vi "Periodic Tasks.vi"(8 "error in":errorcluster) -> ()   [LabVIEW 2017]
doc: "This VI runs in parallel to other tasks. It can contain as many user-defined periodic loops as you need. These can carry out PID or other sorts of timed response."
uses:
  <vilib>/Rock Robotics/WPI/ThirdParty/Phoenix-LabVIEW/Motor Controller/Controls/CTRE_Phoenix_MotorControl_ControlMode.ctl
  SwerveLibrary/Drive Motors.ctl
  SwerveLibrary/Swerve Motors.ctl
  Pigeon IMU.ctl
  Arm Control/Arm Motor.ctl
  <vilib>/Rock Robotics/WPI/Solenoid/WPI_SolenoidValue.ctl
  Robot Global Data.vi
  <vilib>/Rock Robotics/Network Tables/NT Write String.vi
  <vilib>/Rock Robotics/WPI/Solenoid/WPI_SolenoidSetEnum.vi
  <vilib>/Rock Robotics/WPI/ThirdParty/Phoenix-LabVIEW/Motor Controller/Get/CTRE_Phoenix_MotorController_GetSelectedSensorData.vi
  <vilib>/addons/control/pid/pid.llb/PID (DBL).vi
  <vilib>/Rock Robotics/Network Tables/NT Write Number.vi
  SwerveLibrary/Huskie Swerve.lvlib
  <vilib>/addons/control/pid/NI_PID_pid.lvlib
  <vilib>/Rock Robotics/Network Tables/NT Read Number.vi
  <vilib>/Rock Robotics/Network Tables/NT Read Boolean.vi
panel:
  out "error out":errorcluster
  in  "Output range":cluster{"output high":dbl, "output low":dbl}={"output high"=1.0, "output low"=-1.0} {"output low" format="%.2f"; "output high" format="%.2f"}
  in  "Shoulder PID":bool=TRUE
  in  "Forearm PID":bool=TRUE
  out "Forearm output":dbl=0.13174219660051584
  out "Shoulder output":dbl=0.06477138484803567
  out "Shoulder angle":dbl=-0.16720390587953488
  out "Elbow angle":dbl=-2.556378983011421
  in  "Forearm PID gains":T1={"proportional gain (Kc)"=0.5, "integral time (Ti, min)"=0.0, "derivative time (Td, min)"=0.0}
  in  "Shoulder PID gains":T1={"proportional gain (Kc)"=1.5, "integral time (Ti, min)"=0.0, "derivative time (Td, min)"=0.0} {"derivative time (Td, min)" format="%.3f"; "integral time (Ti, min)" format="%.3f"; "proportional gain (Kc)" format="%.3f"}
  in  "Forearm Cap":dbl=0.4
  in  "Shoulder Cap":dbl=0.8
  # "Arm Controls"
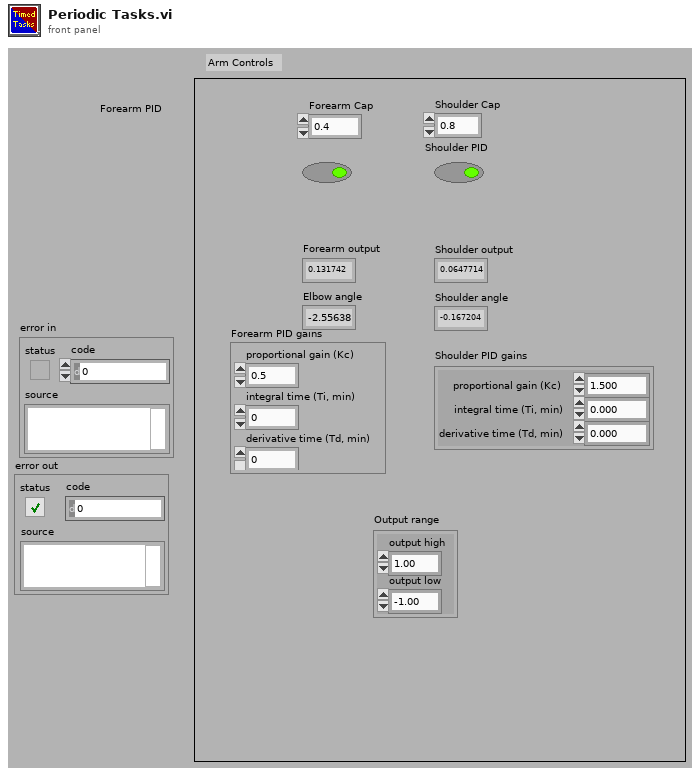
[diagram p1: front panel]
types:
  T1 = cluster{"proportional gain (Kc)":dbl, "integral time (Ti, min)":dbl, "derivative time (Td, min)":dbl}
  T2 = typedef "Pigeon IMU.ctl" = enum16{"Pigeon IMU"}
  T3 = typedef "Huskie Swerve.lvlib/Swerve Motors.ctl" = enum16{"Swerve 1", "Swerve 2", "Swerve 3", "Swerve 4"}
  T4 = typedef "Huskie Swerve.lvlib/Drive Motors.ctl" = enum16{"Drive 1", "Drive 2", "Drive 3", "Drive 4"}
  T5 = typedef "WPI_MotorControlDeviceRef.ctl" = cluster{"DeviceStatus":errorcluster, "Type":T6, "PWM":cluster{"PWM Channel":T7, "DeadBand":T8}, "CAN":cluster{"Device Number":u8, "SetOutput VI Ref":variant, "GetOutput VI Ref":variant, "Enable VI Ref":variant, "Disable VI Ref":variant, "Data":variant}, "Invert":bool, "DIO PWM":cluster{"PWM \"Enable\" Channel":T7, "DIOChannel":T9, "PWM Rate":dbl}}
  T6 = typedef "WPI_MotorControlType.ctl" = enum16{"PWM", "CAN", "DIO PWM"}
  T7 = typedef "FPGA_DIOPWMChannel.ctl" = enum8{"PWM 0", "PWM 1", "PWM 2", "PWM 3", "PWM 4", "PWM 5", "PWM 6", "PWM 7", "PWM 8", "PWM 9", "PWM MXP 0", "PWM MXP 1", "PWM MXP 2", "PWM MXP 3", "PWM MXP 4", "PWM MXP 5", "PWM MXP 6", "PWM MXP 7", "PWM MXP 8", "PWM MXP 9", "Invalid"}
  T8 = typedef "WPI_PWMDeadband.ctl" = cluster{"Name":string, "maxPositivePwm":i32, "minPositivePwm":i32, "centerPwm":i32, "maxNegativePwm":i32, "minNegativePwm":i32, "angularRange":u16}
  T9 = typedef "FPGA_DIOChannel.ctl" = enum8{"DIO 0", "DIO 1", "DIO 2", "DIO 3", "DIO 4", "DIO 5", "DIO 6", "DIO 7", "DIO 8", "DIO 9", "DIO MXP 0", "DIO MXP 1", "DIO MXP 2", "DIO MXP 3", "DIO MXP 4", "DIO MXP 5", "DIO MXP 6", "DIO MXP 7", "DIO MXP 8", "DIO MXP 9", "DIO MXP 10", "DIO MXP 11", "DIO MXP 12", "DIO MXP 13", "DIO MXP 14", "DIO MXP 15", "SPI Port CS1", "SPI Port CS2", "SPI Port CS3", "SPI Port MISO", "SPI Port MOSI", "Invalid"}
  T10 = typedef "CTRE_PigeonIMU_DeviceRef.ctl" = cluster{"DeviceStatus":errorcluster, "Device Number":u8, "Type":T11, "Device ID":u32, "Handle":u64, "UsageFrame":u32, "Library Path":path}
  T11 = typedef "CTRE_PigeonIMU_ConnectionType.ctl" = u32
  T12 = typedef "WPI_DriverStationRobotMode2.ctl" = enum16{"Autonomous Disabled", "Autonomous Enabled", "Teleop Disabled", "Teleop Enabled", "Disconnected", "Finish", "Test Disabled", "Test Enabled", "Emergency Stopped"}
  T13 = cluster{"X":dbl, "Y":dbl, "Z":dbl, "Climber Down":bool, "Climber Up":bool, "X Drive":bool, "Field Relative":bool, "Actuate Grabber":bool, "Inverse Drive":bool}
  T14 = typedef "CTRE_Phoenix_MotorControl_ControlMode.ctl" = u16
  T15 = typedef "WPI_SolenoidValue.ctl" = enum16{"Off", "On", "Forward", "Reverse"}
  T16 = enum16{"Shoulder", "Forearm", "Grabber", "Extra"}[]
  T17 = typedef "Arm Motor.ctl" = enum16{"Shoulder Motor", "Forearm Motor"}
  T18 = typedef "WPI_SolenoidDevRef.ctl" = cluster{"DevStatus":errorcluster, "Pneumatics Control Module":u8, "Forward Solenoid Channel":T19, "Reverse Solenoid Channel":T19}
  T19 = typedef "WPI_SolenoidChannel.ctl" = enum8{"Solenoid 0", "Solenoid 1", "Solenoid 2", "Solenoid 3", "Solenoid 4", "Solenoid 5", "Solenoid 6", "Solenoid 7", "Invalid"}
  T20 = cluster{"Forearm Length":dbl, "Backarm Length":dbl, "Forearm Center of Gravity Length":dbl, "Backarm Center of Gravity Length":dbl, "Weight of Cube":dbl, "Weight of Forearm":dbl, "Weight of Backarm":dbl}
  T21 = cluster{"Forearm importance":dbl, "Backarm importance":dbl}
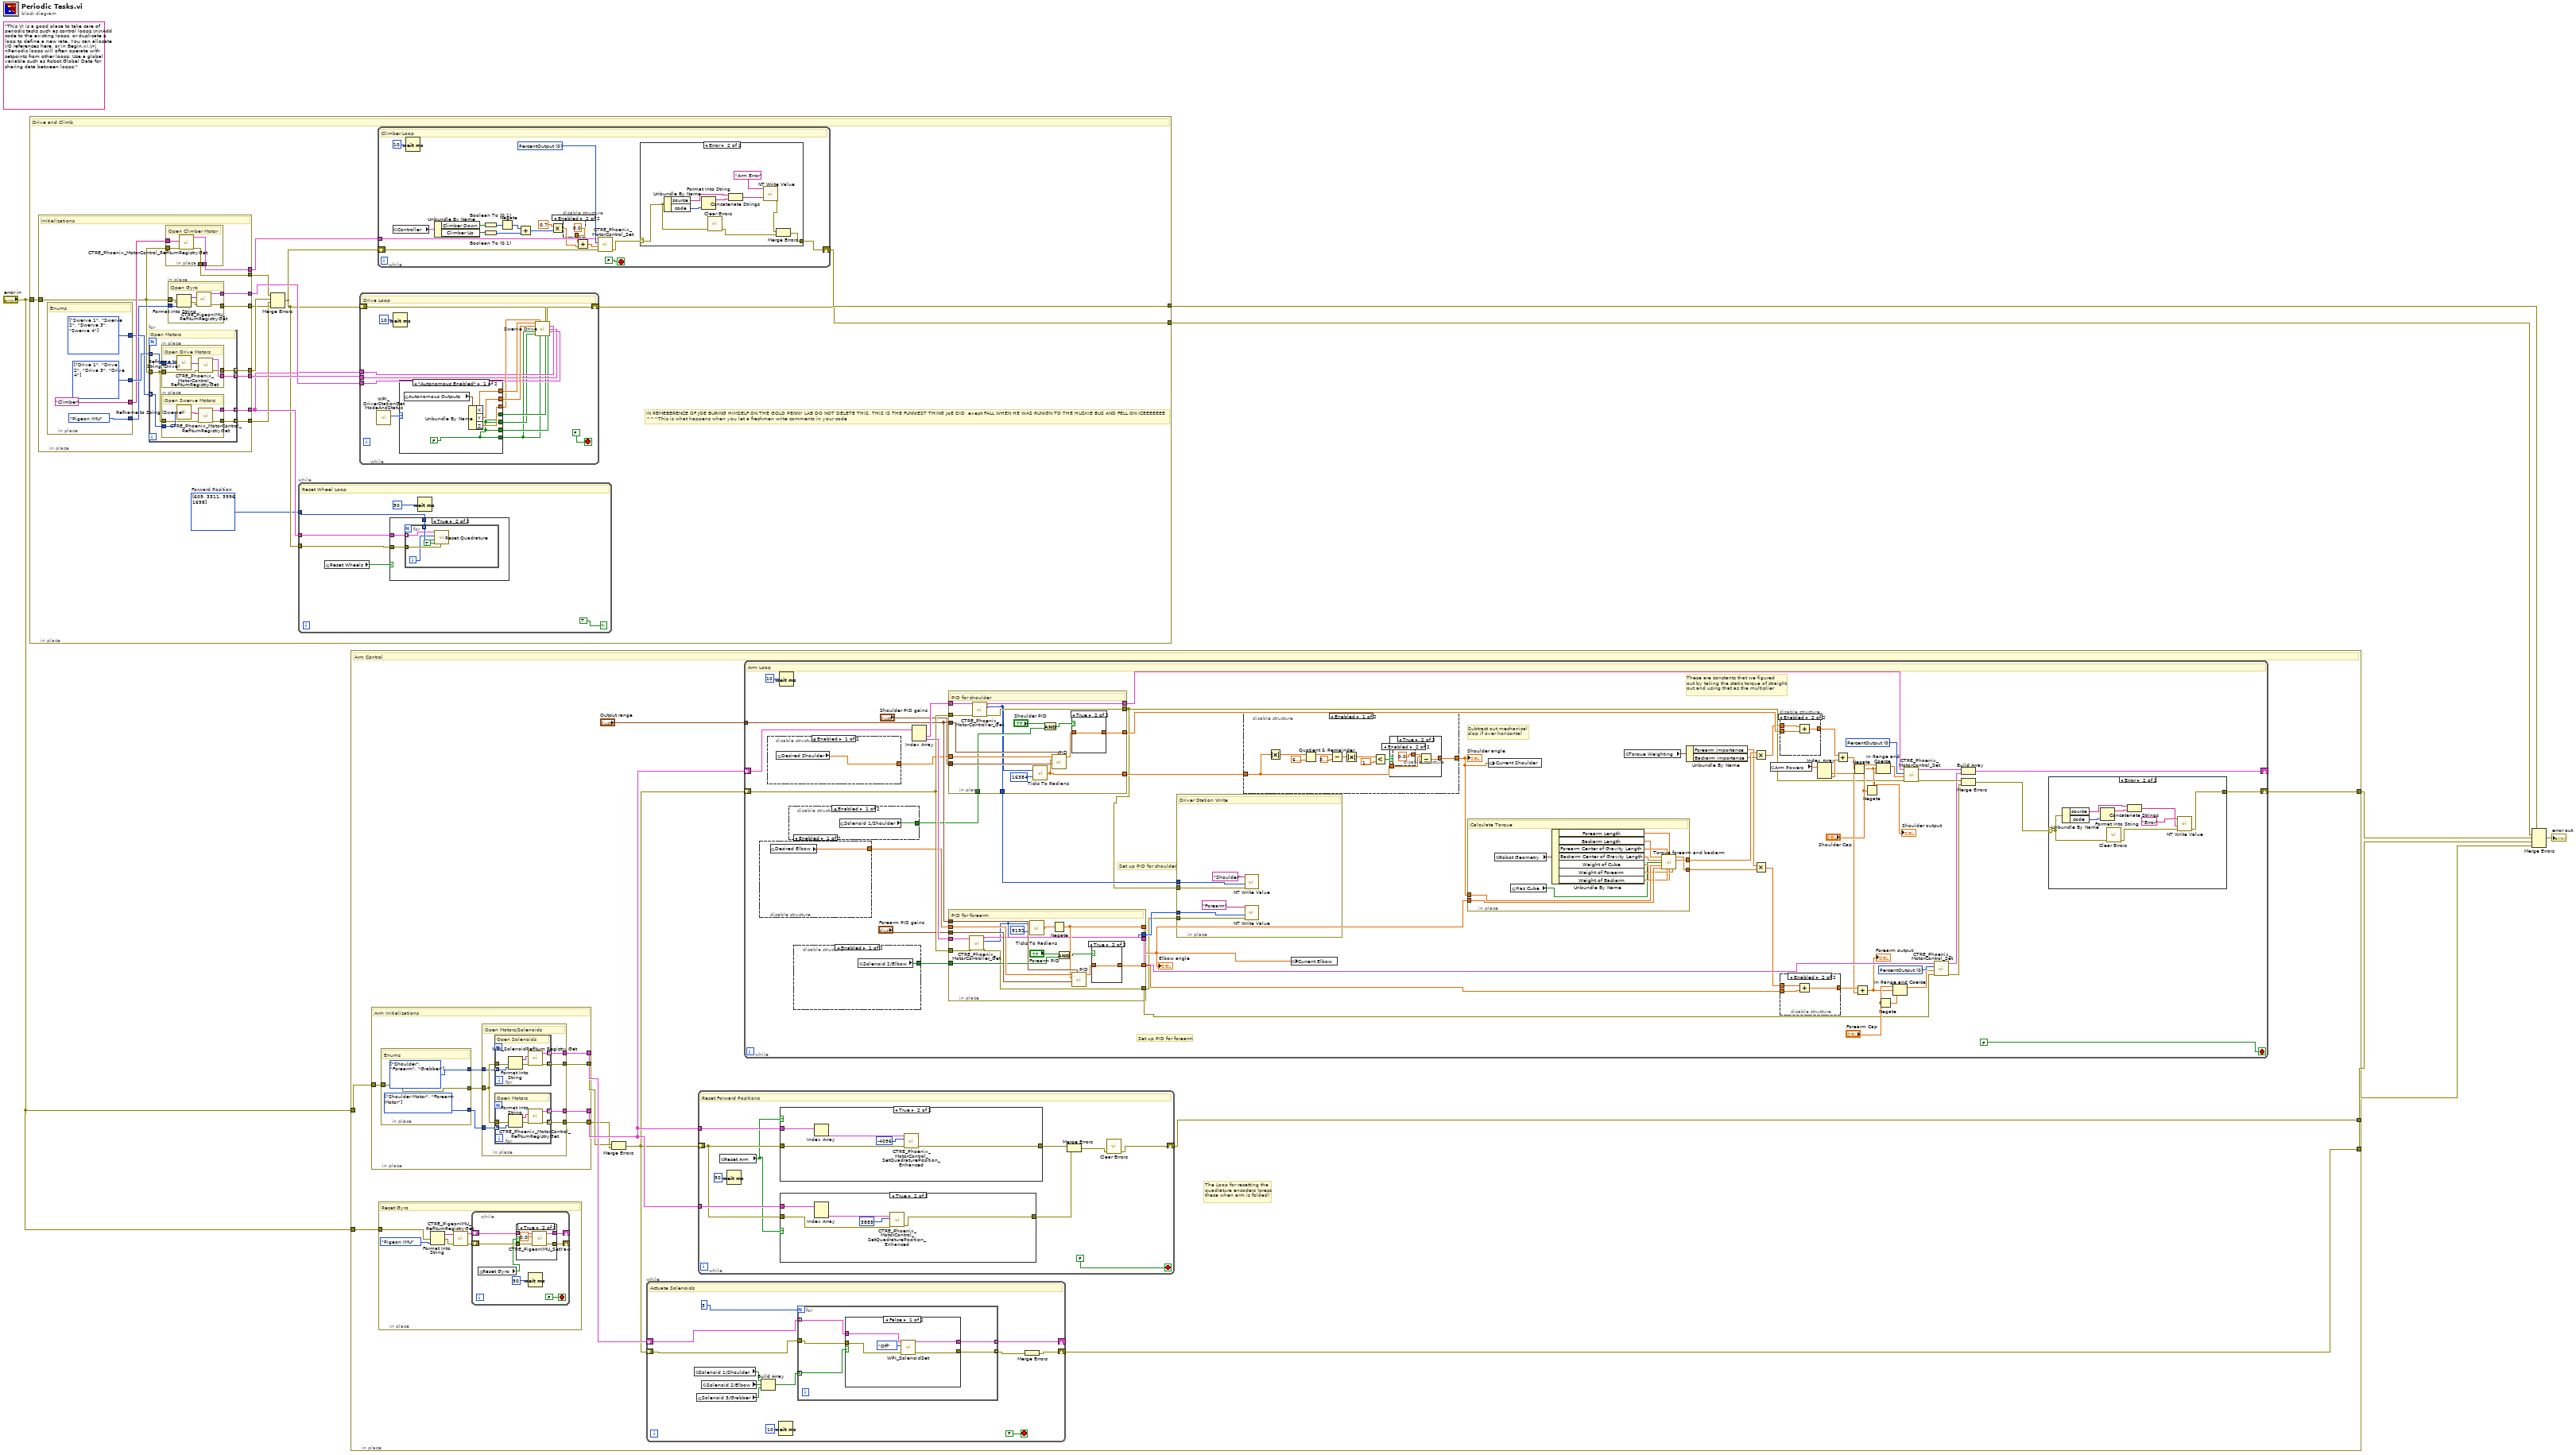
[diagram p0: block diagram]
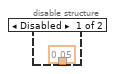
[diagram p3: hidden frame]
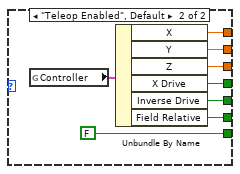
[diagram p5: hidden frame]
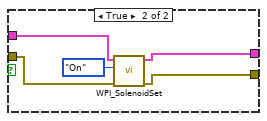
[diagram p7: hidden frame]
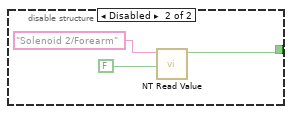
[diagram p10: hidden frame]
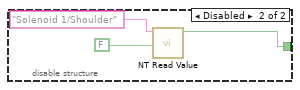
[diagram p11: hidden frame]
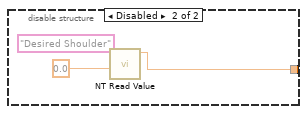
[diagram p12: hidden frame]
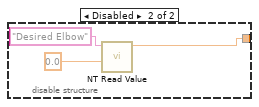
[diagram p13: hidden frame]
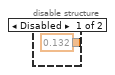
[diagram p16: hidden frame]
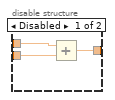
[diagram p18: hidden frame]
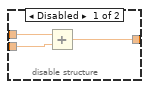
[diagram p19: hidden frame]
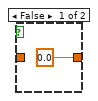
[diagram p20: hidden frame]
diagram:
  (unwired) "This VI is a good place to take care of periodic tasks such as control loops.\n\nAdd code to the existing loops, or duplicate a loop to define a new rate. You can allocate I/O references here, or in Begin.vi.\n\nPeriodic loops will often operate with setpoints from other loops. Use a global variable such as Robot Global Data for sharing data between loops."
  n1 = in-place {
    in-place-border: "error in" -> [w18]
    in-place-border: [w13] -> w7
    in-place-border: [w12] -> w6
    w8 = i32[] [609, 3311, 3996, 1698]  # Forward Position
    # "IN REMEBERENCE OF JOE BURING HIMSELF ON THE GOLD PENNY LAB DO NOT DELETE THIS. THIS IS THE FUNNIEST THING JoE DID  exept FALL WHEN HE WAS RUNIGN TO THE HUSKIE BUS AND FELL ON ICEEEEEEE\n^^^This is what happens when you let a freshmen write comments in your code"
    # "Drive and Climb"
    n2 = in-place {
      in-place-border: [w47] -> w20
      in-place-border: [w46] -> w10
      in-place-border: [w45] -> w19
      in-place-border: [w44] -> w11
      in-place-border: w18 -> [w36]
      in-place-border: [w43] -> w14
      in-place-border: [w42] -> w17
      in-place-border: [w37] -> w16
      in-place-border: [w35] -> w15
      # "Initializations"
      n3 = in-place {
        in-place-border: [w61] -> w41
        in-place-border: ["Climber"] -> w40
        in-place-border: [w59] -> w39
        in-place-border: [Pigeon_IMU."Pigeon IMU" ("Enum")] -> w38
        w59 = T3[] [enum."Swerve 1", enum."Swerve 2", enum."Swerve 3", enum."Swerve 4"] items=["Swerve 1", "Swerve 2", "Swerve 3", "Swerve 4"]
        w61 = T4[] [enum."Drive 1", enum."Drive 2", enum."Drive 3", enum."Drive 4"] items=["Drive 1", "Drive 2", "Drive 3", "Drive 4"]
        # "Enums"
      }
      n4 = for {
        tunnel: w36 -> [w67]
        tunnel: [w68] -> w45 mode=indexing
        tunnel: [w66] -> w47 mode=indexing
        tunnel: [w65] -> w46 mode=indexing
        tunnel: [w64] -> w44 mode=indexing
        tunnel: w41 -> [w63] mode=indexing
        tunnel: w39 -> [w62] mode=indexing
        # "Open Motors"
        n5 = in-place {
          in-place-border: w63 -> [w73]
          in-place-border: [w71] -> w68
          in-place-border: w67 -> [w70]
          in-place-border: [w69] -> w66
          # "Open Drive Motors"
          n6 = call "Refname to String (Drive).vi"("Enum"=w73) -> ("resulting string"=w72:string)
          n7 = call "CTRE_Phoenix_MotorControl_RefNumRegistryGet.vi"("error in (no error)"=w70, "refnum name"=w72) -> ("error out"=w69:errorcluster, "PhoenixMotorControlDevRef"=w71:T5)  [unwired: 8 in]
        }
        n8 = in-place {
          in-place-border: w62 -> [w78]
          in-place-border: w67 -> [w76]
          in-place-border: [w75] -> w65
          in-place-border: [w74] -> w64
          # "Open Swerve Motors"
          n9 = call "Refname to String (Swerve).vi"("Enum"=w78) -> ("String"=w77:string)
          n10 = call "CTRE_Phoenix_MotorControl_RefNumRegistryGet.vi"("error in (no error)"=w76, "refnum name"=w77) -> ("error out"=w75:errorcluster, "PhoenixMotorControlDevRef"=w74:T5)  [unwired: 8 in]
        }
      }
      n11 = in-place {
        in-place-border: w36 -> [w57]
        in-place-border: [w56] -> w43
        in-place-border: [w55] -> w42
        in-place-border: w40 -> [w54]
        # "Open Climber Motor"
        n12 = call "CTRE_Phoenix_MotorControl_RefNumRegistryGet.vi"("error in (no error)"=w57, "refnum name"=w54) -> ("error out"=w56:errorcluster, "PhoenixMotorControlDevRef"=w55:T5)  [unwired: 8 in]
      }
      n13 = in-place {
        in-place-border: w38 -> [w53]
        in-place-border: [w51] -> w37
        in-place-border: w36 -> [w50]
        in-place-border: [w48] -> w35
        # "Open Gyro"
        n14 = Format Into String(error in=w50, w53) -> (resulting string=w52:string, error out=w49:errorcluster)  [unwired: 2 in]
        n15 = call "CTRE_PigeonIMU_RefNumRegistryGet.vi"("error in (no error)"=w49, "refnum name"=w52) -> ("error out"=w48:errorcluster, "PigeonIMUDevRef"=w51:T10)  [unwired: 8 in]
      }
    }
    n16 = Merge Errors(w14, w20, w10, w15) -> (w9:errorcluster)
    n17 = while {
      tunnel: w11 -> [w23]
      tunnel: w9 -> [w25]
      tunnel: w8 -> [w24]
      stop <- TRUE continue-if-true
      # "Reset Wheel Loop"
      n18 = global read "Robot Global Data.vi" "Reset Wheels"() -> (w22:bool)
      n19 = case shown="True" w22 {
        tunnel: w25 -> [_ w29]
        tunnel: w24 -> [_ w28]
        tunnel: w23 -> [_ w27]
        frame False {
        }
        frame True {
          n20 = for {
            tunnel: w29 -> [w34]
            tunnel: w28 -> [w32] mode=indexing
            tunnel: w27 -> [w30] mode=indexing
            i -> [w31]
            n21 = call "Reset Quadrature.vi"("error in"=w34, "Reverse?"=TRUE, "Forward Position"=w32, "Module Number"=w31, "CAN Talon SRX Ref"=w30) -> ()  [unwired: 5 in, 2 out]
          }
        }
      }
      n22 = Wait (ms)(milliseconds to wait=50) -> ()  [unwired: 1 out]
    }
    n23 = while {
      tunnel: w19 -> [w114]
      tunnel: w11 -> [w116]
      tunnel: w16 -> [w115]
      shift-right: [w117] -> w12
      shift-left: w9 -> [w118]
      stop <- FALSE stop-if-true
      # "Drive Loop"
      n24 = call <vilib>:"WPI_DriverStationGetModeAndStatus.vi"() -> ("Robot Mode"=w109:T12)  [unwired: 10 in, 1 out]
      n25 = Wait (ms)(milliseconds to wait=u32 10) -> ()  [unwired: 1 out]
      n26 = case shown="\"Autonomous Enabled\"" w109 {
        tunnel: [w125 w135] -> w121
        tunnel: [w126 w134] -> w120
        tunnel: [w127 w133] -> w119
        tunnel: [w124 w132] -> w113
        tunnel: [w124 w131] -> w112
        tunnel: [w124 w130] -> w111
        tunnel: [w124 FALSE] -> w110
        frame "Autonomous Enabled" {
          w124 = FALSE
          n27 = global read "Robot Global Data.vi" "Autonomous Outputs"() -> (w128:cluster{"X":dbl, "Y":dbl, "Z":dbl})
          n28 = Unbundle By Name(w128) -> ("X"=w125:dbl, "Y"=w126:dbl, "Z"=w127:dbl)
        }
        frame "Teleop Enabled", Default {
          n29 = global read "Robot Global Data.vi" "Controller"() -> (w136:T13)
          n30 = Unbundle By Name(w136) -> ("X"=w135:dbl, "Y"=w134:dbl, "Z"=w133:dbl, "X Drive"=w132:bool, "Inverse Drive"=w130:bool, "Field Relative"=w131:bool)
        }
      }
      n31 = call "Swerve Drive.vi"("X"=w121, "Z"=w119, "error in"=w118, "Y"=w120, "Swerve Dev Ref"=w116, "Drive Dev Ref"=w114, "Straight Drive"=w110, "PigeonIMUDevRef"=w115, "Reverse Drive"=w111, "Low Sensitivity"=w110, "X Drive"=w113, "Field Relative Active"=w112) -> ("error out"=w117:errorcluster)  [unwired: 3 in]
    }
    n32 = while {
      tunnel: w17 -> [w87]
      shift-right: [w82] -> w13
      shift-left: w9 -> [w88]
      stop <- FALSE stop-if-true
      w96 = T14 0 items=["PercentOutput"=0, "Position"=1, "Velocity"=2, "Current"=3, "Follower"=5, "MotionProfile"=6, "MotionMagic"=7, "MotionMagicArc"=8, "MotionProfileArc"=10, "Disabled"=15] ("Control Mode")
      # "Climber Loop"
      n33 = global read "Robot Global Data.vi" "Controller"() -> (w95:T13)
      n34 = Wait (ms)(milliseconds to wait=10) -> ()  [unwired: 1 out]
      n35 = Unbundle By Name(w95) -> ("Climber Down"=w94:bool, "Climber Up"=w93:bool)
      n36 = Boolean To (0,1)(Boolean=w94) -> (0, 1=w92:i16)
      n37 = Boolean To (0,1)(Boolean=w93) -> (0, 1=w90:i16)
      n38 = Negate(x=w92) -> (-x=w91:i16)
      n39 = Add(x=w91, y=w90) -> (x+y=w85:i16)
      n40 = Multiply(x=0.7, y=w85) -> (x*y=w81:dbl)
      n41 = disable-structure shown="Enabled" {
        disable-tunnel: [0.05 0.0] -> w80
        frame Disabled {
        }
        frame Enabled {
        }
      }
      n42 = Add(x=w80, y=w81) -> (x+y=w79:dbl)
      n43 = call "CTRE_Phoenix_MotorControl_Set.vi"("error in (no error)"=w88, "Output"=w79, "Control Mode"=w96, "PhoenixMotorControlDevRef"=w87) -> ("error out"=w83:errorcluster)  [unwired: 6 in, 1 out]
      n44 = case shown="Error" w83 {
        selector: w83 -> [w99 w104]
        tunnel: [w99 w100] -> w82
        frame No Error {
        }
        frame Error {
          n45 = Unbundle By Name(w104) -> ("source"=w106:string, "code"=w108:i32)
          n46 = Format Into String(w108) -> (resulting string=w107:string)  [unwired: 3 in, 1 out]
          n47 = call <vilib>:"Clear Errors.vi"("error in (no error)"=w104) -> ("error out"=w102:errorcluster)  [unwired: 5 in, 1 out]
          n48 = Concatenate Strings(w106, w107) -> (w103:string)
          n49 = call-poly <vilib>:"NT Write Value.vi"("String"=w103, "Name"="Arm Error") -> ("error out"=w101:errorcluster)  [unwired: 9 in]
          n50 = Merge Errors(w101, w102) -> (w100:errorcluster)
        }
      }
    }
  }
  n51 = in-place "In Place Element Structure" {
    in-place-border: "error in" -> [w144]
    in-place-border: [w140] -> w5
    in-place-border: [w139] -> w4
    in-place-border: [w138] -> w3
    in-place-border: "error in" -> [w137]
    # "The Loop for resetting the\nquadrature encoders (press\nthese when arm is folded)"
    # "Arm Control"
    n52 = in-place {
      in-place-border: [w174] -> w142
      in-place-border: [w173] -> w146
      in-place-border: [w172] -> w145
      in-place-border: [w171] -> w143
      in-place-border: w144 -> [w169]
      # "Arm Initializations"
      n53 = in-place {
        in-place-border: [w197] -> w175
        in-place-border: [w196] -> w170
        in-place-border: w169 -> [w195]
        in-place-border: [w195] -> w168
        w196 = T16 [enum."Shoulder", enum."Forearm", enum."Grabber"] items=["Shoulder", "Forearm", "Grabber", "Extra"]
        w197 = T17[] [enum."Shoulder Motor", enum."Forearm Motor"] items=["Shoulder Motor", "Forearm Motor"]
        # "Enums"
      }
      n54 = in-place {
        in-place-border: w175 -> [w182]
        in-place-border: [w181] -> w174
        in-place-border: [w180] -> w173
        in-place-border: [w179] -> w172
        in-place-border: [w178] -> w171
        in-place-border: w168 -> [w177]
        in-place-border: w170 -> [w176]
        # "Open Motors/Solenoids"
        n55 = for {
          tunnel: w176 -> [w194] mode=indexing
          tunnel: w177 -> [w193]
          tunnel: [w190] -> w179 mode=indexing
          tunnel: [w189] -> w178 mode=indexing
          # "Open Solenoids"
          n56 = Format Into String(error in=w193, w194) -> (resulting string=w192:string, error out=w191:errorcluster)  [unwired: 2 in]
          n57 = call <vilib>:"WPI_SolenoidRefNum Registry Get.vi"("error in (no error)"=w191, "refnum name"=w192) -> ("error out"=w189:errorcluster, "SolenoidDevRef"=w190:T18)  [unwired: 8 in]
        }
        n58 = for {
          tunnel: w182 -> [w187] mode=indexing
          tunnel: [w186] -> w180 mode=indexing
          tunnel: [w185] -> w181 mode=indexing
          tunnel: w177 -> [w183]
          # "Open Motors"
          n59 = Format Into String(error in=w183, w187) -> (resulting string=w188:string, error out=w184:errorcluster)  [unwired: 2 in]
          n60 = call "CTRE_Phoenix_MotorControl_RefNumRegistryGet.vi"("error in (no error)"=w184, "refnum name"=w188) -> ("error out"=w185:errorcluster, "PhoenixMotorControlDevRef"=w186:T5)  [unwired: 8 in]
        }
      }
    }
    n61 = in-place "In Place Element Structure" {
      in-place-border: w137 -> [w148]
      # "Reset Gyro"
      n62 = Format Into String(error in=w148, Pigeon_IMU."Pigeon IMU" ("Enum")) -> (resulting string=w152:string, error out=w149:errorcluster)  [unwired: 2 in]
      n63 = call "CTRE_PigeonIMU_RefNumRegistryGet.vi"("error in (no error)"=w149, "refnum name"=w152) -> ("error out"=w151:errorcluster, "PigeonIMUDevRef"=w150:T10)  [unwired: 8 in]
      n64 = while {
        shift-right: [w158] -> _
        shift-left: w150 -> [w159]
        shift-right: [w157] -> _
        shift-left: w151 -> [w160]
        stop <- FALSE stop-if-true
        n65 = global read "Robot Global Data.vi" "Reset Gyro"() -> (w154:bool)
        n66 = case shown="True" w154 {
          tunnel: w160 -> [w161 w167]
          tunnel: w159 -> [w162 w166]
          tunnel: [w162 w164] -> w158
          tunnel: [w161 w163] -> w157
          frame False {
          }
          frame True {
            n67 = call <vilib>:"CTRE_PigeonIMU_SetYaw.vi"("error in (no error)"=w167, "Value"=0.0, "PigeonIMUDevRef"=w166) -> ("error out"=w163:errorcluster, "PigeonIMUDevRef"=w164:T10)  [unwired: 7 in]
          }
        }
        n68 = Wait (ms)(milliseconds to wait=50) -> ()  [unwired: 1 out]
      }
    }
    n69 = Merge Errors(w143, w142) -> (w141:errorcluster)
    n70 = while {
      shift-right: [w203] -> _
      shift-left: w145 -> [w207]
      shift-right: [w198] -> w138
      shift-left: w141 -> [w205]
      stop <- FALSE stop-if-true
      # "Actuate Solenoids"
      n71 = global read "Robot Global Data.vi" "Solenoid 1/Shoulder"() -> (w202:bool)
      n72 = global read "Robot Global Data.vi" "Solenoid 3/Grabber"() -> (w200:bool)
      n73 = global read "Robot Global Data.vi" "Solenoid 2/Elbow"() -> (w201:bool)
      n74 = Build Array(w202, w201, w200) -> (w204:bool[])
      n75 = Wait (ms)(milliseconds to wait=u32 10) -> ()  [unwired: 1 out]
      n76 = for {
        N: 3 -> [_]
        tunnel: w207 -> [w212] mode=indexing
        tunnel: w205 -> [w213]
        tunnel: w204 -> [w214] mode=indexing
        tunnel: [w211] -> w203 mode=indexing
        tunnel: [w210] -> w199 mode=indexing
        n77 = case shown="False" w214 {
          tunnel: w213 -> [w218 w224]
          tunnel: w212 -> [w217 w222]
          tunnel: [w216 w221] -> w211
          tunnel: [w215 w220] -> w210
          frame False {
            n78 = call-poly <vilib>:"WPI_SolenoidSet.vi"("error in (no error)"=w218, "Value"=WPI_SolenoidValue."Off", "SolenoidDevRef"=w217) -> ("error out"=w215:errorcluster, "SolenoidDevRef"=w216:T18)  [unwired: 7 in]
          }
          frame True {
            n79 = call-poly <vilib>:"WPI_SolenoidSet.vi"("error in (no error)"=w224, "Value"=WPI_SolenoidValue."On", "SolenoidDevRef"=w222) -> ("error out"=w220:errorcluster, "SolenoidDevRef"=w221:T18)  [unwired: 7 in]
          }
        }
      }
      n80 = Merge Errors(w199) -> (w198:errorcluster)
    }
    n81 = while {
      tunnel: w146 -> [w233]
      shift-right: [w225] -> w139
      shift-left: w141 -> [w230]
      tunnel: w146 -> [w232]
      stop <- FALSE stop-if-true
      # "Reset Forward Positions"
      n82 = global read "Robot Global Data.vi" "Reset Arm"() -> (w227:bool)
      n83 = Wait (ms)(milliseconds to wait=u32 50) -> ()  [unwired: 1 out]
      n84 = case shown="True" w227 {
        tunnel: w233 -> [_ w246]
        tunnel: w230 -> [w241 w245]
        tunnel: [w241 w243] -> w228
        frame False {
        }
        frame True {
          n85 = Index Array(array=w246) -> (element=w244:T5)  [unwired: 1 in]
          n86 = call <vilib>:"CTRE_Phoenix_MotorControl_SetQuadraturePosition_Enhanced.vi"("error in (no error)"=w245, "New Position"=-4096, "PhoenixMotorControlDevRef"=w244) -> ("error out"=w243:errorcluster)  [unwired: 7 in, 1 out]
        }
      }
      n87 = case shown="True" w227 {
        tunnel: w232 -> [_ w240]
        tunnel: w230 -> [w235 w238]
        tunnel: [w235 w237] -> w229
        frame False {
        }
        frame True {
          n88 = Index Array(array=w240) -> (element #2=w239:T5)  [unwired: 2 in, 1 out]
          n89 = call <vilib>:"CTRE_Phoenix_MotorControl_SetQuadraturePosition_Enhanced.vi"("error in (no error)"=w238, "New Position"=3885, "PhoenixMotorControlDevRef"=w239) -> ("error out"=w237:errorcluster)  [unwired: 7 in, 1 out]
        }
      }
      n90 = Merge Errors(w228, w229) -> (w226:errorcluster)
      n91 = call <vilib>:"Clear Errors.vi"("error in (no error)"=w226) -> ("error out"=w225:errorcluster)  [unwired: 5 in, 1 out]
    }
    n92 = while {
      tunnel: "Output range" -> [w289]
      shift-right: [w291] -> _
      shift-left: w146 -> [w299]
      shift-right: [w249] -> w140
      shift-left: w141 -> [w286]
      stop <- FALSE stop-if-true
      w288 = T14 0 items=["PercentOutput"=0, "Position"=1, "Velocity"=2, "Current"=3, "Follower"=5, "MotionProfile"=6, "MotionMagic"=7, "MotionMagicArc"=8, "MotionProfileArc"=10, "Disabled"=15] ("Control Mode")
      w295 = T14 0 items=["PercentOutput"=0, "Position"=1, "Velocity"=2, "Current"=3, "Follower"=5, "MotionProfile"=6, "MotionMagic"=7, "MotionMagicArc"=8, "MotionProfileArc"=10, "Disabled"=15] ("Control Mode")
      # "Subtract out mechanical\nslop if over horizontal"
      # "Set up PID for shoulder"
      # "These are constants that we figured\nout by taking the static torque of straight\nout and using that as the multiplier"
      # "Set up PID for forearm"
      # "Arm Loop"
      n93 = disable-structure shown="Enabled" {
        disable-tunnel: [w313 w314] -> w281
        frame Enabled {
          n94 = global read "Robot Global Data.vi" "Desired Elbow"() -> (w313:dbl)
        }
        frame Disabled {
          n95 = call-poly <vilib>:"NT Read Value.vi"("Default Value"=0.0, "Name"="Desired Elbow") -> ("Numeric"=w314:dbl)  [unwired: 8 in, 1 out]
        }
      }
      n96 = disable-structure shown="Enabled" {
        disable-tunnel: [w309 w310] -> w282
        frame Enabled {
          n97 = global read "Robot Global Data.vi" "Desired Shoulder"() -> (w309:dbl)
        }
        frame Disabled {
          n98 = call-poly <vilib>:"NT Read Value.vi"("Default Value"=0.0, "Name"="Desired Shoulder") -> ("Numeric"=w310:dbl)  [unwired: 8 in, 1 out]
        }
      }
      n99 = Wait (ms)(milliseconds to wait=10) -> ()  [unwired: 1 out]
      n100 = disable-structure shown="Enabled" {
        disable-tunnel: [w305 w308] -> w258
        frame Enabled {
          n101 = global read "Robot Global Data.vi" "Solenoid 1/Shoulder"() -> (w305:bool)
        }
        frame Disabled {
          n102 = call-poly <vilib>:"NT Read Value.vi"("Default Value"=FALSE, "Name"="Solenoid 1/Shoulder") -> ("Boolean"=w308:bool)  [unwired: 8 in, 1 out]
        }
      }
      n103 = disable-structure shown="Enabled" {
        disable-tunnel: [w301 w303] -> w259
        frame Enabled {
          n104 = global read "Robot Global Data.vi" "Solenoid 2/Elbow"() -> (w301:bool)
        }
        frame Disabled {
          n105 = call-poly <vilib>:"NT Read Value.vi"("Default Value"=FALSE, "Name"="Solenoid 2/Forearm") -> ("Boolean"=w303:bool)  [unwired: 8 in, 1 out]
        }
      }
      n106 = Index Array(array=w299) -> (element #1=w298:T5, element #2=w290:T5)  [unwired: 2 in]
      n107 = in-place "In Place Element Structure" {
        in-place-border: "Shoulder PID gains" -> [w406]
        in-place-border: w289 -> [w405]
        in-place-border: w298 -> [w396]
        in-place-border: w286 -> [w393]
        in-place-border: [w403] -> w297
        in-place-border: [w394] -> w252
        in-place-border: [w395] -> w296
        in-place-border: [w397] -> w267
        in-place-border: w282 -> [w404]
        in-place-border: w258 -> [w399]
        in-place-border: [w392] -> w253
        # "PID for shoulder"
        n108 = call-poly "CTRE_Phoenix_MotorController_Get.vi"("PhoenixMotorControlDevRef"=w396, "error in"=w393) -> ("PhoenixMotorControlDevRef"=w395:T5, "Position (Raw Sensor Units)"=w392:i32, "error out"=w394:errorcluster)  [unwired: 10 in, 1 out]
        n109 = call "Ticks To Radians.vi"("Ticks/Rev"=16384, "Ticks"=w392) -> ("Radians"=w397:dbl)
        n110 = And(x="Shoulder PID", y=w399) -> (x .and. y?=w401:bool)
        n111 = call-poly <vilib>:"PID.vi"("output range"=w405, "PID gains"=w406, "process variable"=w397, "setpoint"=w404) -> ("output"=w402:dbl)  [unwired: 6 in, 1 out]
        n112 = case shown="True" w401 {
          tunnel: [0.0 w408] -> w403
          tunnel: w402 -> [_ w408]
          frame False {
          }
          frame True {
          }
        }
      }
      n113 = in-place "In Place Element Structure" {
        in-place-border: w290 -> [w365]
        in-place-border: w289 -> [w376]
        in-place-border: [w372] -> w287
        in-place-border: [w363] -> w251
        in-place-border: w286 -> [w364]
        in-place-border: [w362] -> w283
        in-place-border: w281 -> [w375]
        in-place-border: "Forearm PID gains" -> [w374]
        in-place-border: [w371] -> w257
        in-place-border: w259 -> [w368]
        in-place-border: [w361] -> w254
        # "PID for forearm"
        n114 = call-poly "CTRE_Phoenix_MotorController_Get.vi"("PhoenixMotorControlDevRef"=w365, "error in"=w364) -> ("PhoenixMotorControlDevRef"=w362:T5, "Position (Raw Sensor Units)"=w361:i32, "error out"=w363:errorcluster)  [unwired: 10 in, 1 out]
        n115 = call "Ticks To Radians.vi"("Ticks/Rev"=8192, "Ticks"=w361) -> ("Radians"=w367:dbl)
        n116 = Negate(x=w367) -> (-x=w371:dbl)
        n117 = And(x="Forearm PID", y=w368) -> (x .and. y?=w369:bool)
        n118 = call-poly <vilib>:"PID.vi"("output range"=w376, "PID gains"=w374, "process variable"=w371, "setpoint"=w375) -> ("output"=w373:dbl)  [unwired: 6 in, 1 out]
        n119 = case shown="True" w369 {
          tunnel: w373 -> [_ w378]
          tunnel: [0.0 w378] -> w372
          frame False {
          }
          frame True {
          }
        }
      }
      "Elbow angle" <- w257
      n120 = in-place {
        in-place-border: w254 -> [w331]
        in-place-border: w253 -> [w328]
        in-place-border: w252 -> [w327]
        in-place-border: w251 -> [w326]
        # "Driver Station Write"
        n121 = call-poly <vilib>:"NT Write Value.vi"("error in"=w327, "Numeric"=w328, "Name"="Shoulder") -> ()  [unwired: 8 in, 1 out]
        n122 = call-poly <vilib>:"NT Write Value.vi"("error in"=w326, "Numeric"=w331, "Name"="Forearm") -> ()  [unwired: 8 in, 1 out]
      }
      n123 = disable-structure shown="Enabled" {
        disable-tunnel: w267 -> [w338 w348]
        disable-tunnel: [w332 w348] -> w256
        frame Enabled {
          n124 = Absolute Value(x=w338) -> (abs(x)=w339:dbl)
          n125 = Quotient & Remainder(x=w339, y=6.283185307179586) -> (x-y*floor(x/y)=w337:dbl)  [unwired: 1 out]
          n126 = Subtract(x=w337, y=3.141592653589793) -> (x-y=w335:dbl)
          n127 = Absolute Value(x=w335) -> (abs(x)=w334:dbl)
          n128 = Less?(x=w334, y=1.5707963267948966) -> (x < y?=w341:bool)
          n129 = case shown="True" w341 {
            tunnel: w338 -> [w342 w344]
            tunnel: [w342 w345] -> w332
            frame False {
            }
            frame True {
              n130 = disable-structure shown="Enabled" {
                disable-tunnel: [0.132 0.0] -> w343
                frame Disabled {
                }
                frame Enabled {
                }
              }
              n131 = Subtract(x=w344, y=w343) -> (x-y=w345:dbl)
            }
          }
        }
        frame Disabled {
        }
      }
      "Shoulder angle" <- w256
      n132 = global write "Robot Global Data.vi" "Current Elbow"(w257) -> ()
      n133 = in-place "In Place Element Structure" {
        in-place-border: w256 -> [w391]
        in-place-border: w257 -> [w390]
        in-place-border: [w389] -> w279
        in-place-border: [w388] -> w275
        # "Calculate Torque"
        n134 = global read "Robot Global Data.vi" "Robot Geometry"() -> (w387:T20)
        n135 = global read "Robot Global Data.vi" "Has Cube"() -> (w379:bool)
        n136 = Unbundle By Name(w387) -> ("Forearm Length"=w386:dbl, "Backarm Length"=w384:dbl, "Forearm Center of Gravity Length"=w385:dbl, "Backarm Center of Gravity Length"=w383:dbl, "Weight of Cube"=w382:dbl, "Weight of Forearm"=w381:dbl, "Weight of Backarm"=w380:dbl)
        n137 = call "Torque forearm and backarm.vi"("Backarm Length"=w384, "Forearm Center of Gravity Length"=w385, "Forearm Length"=w386, "Backarm Center of Gravity Length"=w383, "If has block"=w379, "Alpha"=w391, "Beta"=w390, "Weight of cube"=w382, "Weight of Backarm"=w380, "Weight of Forearm"=w381) -> ("Torque of forearm"=w388:dbl, "Torque of shoulder"=w389:dbl)  [unwired: 4 in]
      }
      n138 = global write "Robot Global Data.vi" "Current Shoulder"(w256) -> ()
      n139 = global read "Robot Global Data.vi" "Torque Weighting"() -> (w280:T21)
      n140 = Unbundle By Name(w280) -> ("Forearm importance"=w276:dbl, "Backarm importance"=w278:dbl)
      n141 = Multiply(x=w279, y=w278) -> (x*y=w277:dbl)
      n142 = Multiply(x=w276, y=w275) -> (x*y=w274:dbl)
      n143 = global read "Robot Global Data.vi" "Arm Powers"() -> (w273:dbl[])
      n144 = disable-structure shown="Enabled" {
        disable-tunnel: w297 -> [w351 w352]
        disable-tunnel: [w350 w354] -> w271
        disable-tunnel: w277 -> [w349 w353]
        frame Disabled {
          n145 = Add(x=w349, y=w351) -> (x+y=w350:dbl)
        }
        frame Enabled {
          n146 = Add(x=w353, y=w352) -> (x+y=w354:dbl)
        }
      }
      n147 = disable-structure shown="Enabled" {
        disable-tunnel: [w357 w358] -> w272
        disable-tunnel: w287 -> [w356 w359]
        disable-tunnel: w274 -> [w355 w360]
        frame Disabled {
          n148 = Add(x=w355, y=w356) -> (x+y=w357:dbl)
        }
        frame Enabled {
          n149 = Add(x=w360, y=w359) -> (x+y=w358:dbl)
        }
      }
      n150 = Index Array(array=w273) -> (element #1=w255:dbl, element #2=w270:dbl)  [unwired: 2 in]
      n151 = Add(x=w271, y=w270) -> (x+y=w260:dbl)
      n152 = Negate(x=w260) -> (-x=w248:dbl)
      "Shoulder output" <- w248
      n153 = Add(x=w272, y=w255) -> (x+y=w247:dbl)
      "Forearm output" <- w247
      n154 = Negate(x="Shoulder Cap") -> (-x=w261:dbl)
      n155 = In Range and Coerce(upper limit="Shoulder Cap", x=w248, lower limit=w261) -> (coerced(x)=w268:dbl)  [unwired: 1 out]
      n156 = Negate(x="Forearm Cap") -> (-x=w264:dbl)
      n157 = In Range and Coerce(upper limit="Forearm Cap", x=w247, lower limit=w264) -> (coerced(x)=w269:dbl)  [unwired: 1 out]
      n158 = call "CTRE_Phoenix_MotorControl_Set.vi"("error in (no error)"=w252, "Output"=w268, "Control Mode"=w295, "PhoenixMotorControlDevRef"=w296) -> ("error out"=w293:errorcluster, "PhoenixMotorControlDevRef"=w292:T5)  [unwired: 6 in]
      n159 = call "CTRE_Phoenix_MotorControl_Set.vi"("error in (no error)"=w251, "Output"=w269, "Control Mode"=w288, "PhoenixMotorControlDevRef"=w283) -> ("error out"=w285:errorcluster, "PhoenixMotorControlDevRef"=w284:T5)  [unwired: 6 in]
      n160 = Build Array(w292, w284) -> (w291:T5[])
      n161 = Merge Errors(w293, w285) -> (w250:errorcluster)
      n162 = case shown="Error" w250 {
        selector: w250 -> [w317 w319]
        tunnel: [w317 w320] -> w249
        frame No Error {
        }
        frame Error {
          n163 = Unbundle By Name(w319) -> ("source"=w322:string, "code"=w324:i32)
          n164 = Format Into String(w324) -> (resulting string=w323:string)  [unwired: 3 in, 1 out]
          n165 = call <vilib>:"Clear Errors.vi"("error in (no error)"=w319) -> ("error out"=w318:errorcluster)  [unwired: 5 in, 1 out]
          n166 = Concatenate Strings(w322, w323) -> (w321:string)
          n167 = call-poly <vilib>:"NT Write Value.vi"("error in"=w318, "String"=w321, "Name"="Error") -> ("error out"=w320:errorcluster)  [unwired: 8 in]
        }
      }
    }
  }
  n168 = Merge Errors(w7, w6, w5, w4, w3) -> (→"error out":errorcluster)
